vi "Get All Frame and Signal Names.vi"(0 "XNET Frames":refnum<k21>[](array[refnum]), 11 "error in":errorcluster) -> (4 "Frame Names":string[](array[string]), 6 "Number of Frames":i32, 8 "Signal Names":string[][](array[string]), 10 "Number of Signals":i32[](array[numeric]), 15 "error out":errorcluster)   [LabVIEW 2015]
uses:
  <resource>/objmgr/xnet.rc
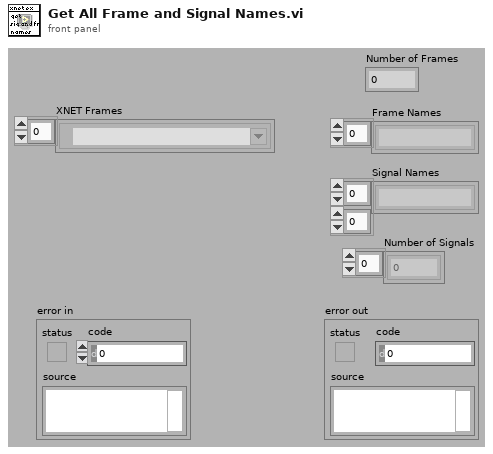
[diagram p1: front panel]
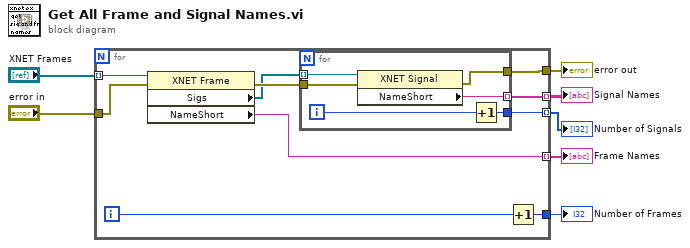
[diagram p0: block diagram]
diagram:
  n1 = for {
    tunnel: "XNET Frames" -> [w11] mode=indexing
    tunnel: [w17] -> w4
    tunnel: "error in" -> [w10]
    tunnel: [w15] -> w5 mode=indexing
    tunnel: [w8] -> w6 mode=indexing
    tunnel: [w14] -> w2 mode=indexing
    tunnel: [w13] -> w1
    i -> [w12]
    n2 = property class="XNET Frame"(reference=w11, error in=w10) -> (error out=w16:errorcluster, "Sigs"=w9:refnum<k21>[], "NameShort"=w8:string)  [unwired: 1 out]
    n3 = for {
      tunnel: w9 -> [w19] mode=indexing
      tunnel: [w23] -> w17
      tunnel: w16 -> [w18]
      tunnel: [w22] -> w15 mode=indexing
      tunnel: [w20] -> w14
      i -> [w21]
      n4 = property class="XNET Signal"(reference=w19, error in=w18) -> (error out=w23:errorcluster, "NameShort"=w22:string)  [unwired: 1 out]
      n5 = Increment(x=w21) -> (x+1=w20:i32)
    }
    n6 = Increment(x=w12) -> (x+1=w13:i32)
  }
  "Frame Names" <- w6
  "Signal Names" <- w5
  "error out" <- w4
  "Number of Frames" <- w1
  "Number of Signals" <- w2
